vi "Taiko_TaggedValueListToStr.vi"(10 "TaggedValueList in":T1 {"Tag" format="%x" items=["NONE"=0, "Locked"=16, "SoftLock"=17, "KeyLock"=18, "Class_IV_Lock"=20, "Interlock"=24, "LaserMode"=32, "LDH_PulsePowerTable"=33, "TriggerMode"=48, "TriggerLevelRaw"=64, "TriggerLevelRawLoLimit"=65, "TriggerLevelRawHiLimit"=66, "TriggerLevel"=72, "TriggerLevelLoLimit"=73, "TriggerLevelHiLimit"=74, "FastGate"=80, "FastGateImp"=96, "SlowGate"=112, "TargetTempRaw"=144, "TargetTempRawLoLimit"=145, "TargetTempRawHiLimit"=146, "CurrentTempRaw"=148, "CaseTempRaw"=149, "TargetTemp"=152, "TargetTempLoLimit"=153, "TargetTempHiLimit"=154, "CurrentTemp"=156, "CaseTemp"=157, "TempScale"=159, "Frequency"=168, "FrequencyLoLimit"=169, "FrequencyHiLimit"=170, "PulsePowerRaw"=176, "PulsePowerRawLoLimit"=177, "PulsePowerRawHiLimit"=178, "PulsePowerPermille"=180, "PulseShape"=181, "PulsePower"=184, "PulsePowerLoLimit"=185, "PulsePowerHiLimit"=186, "PulsePowerNanowatt"=188, "PulsePowerVoltage"=190, "PulseEnergy"=191, "CwPowerRaw"=192, "CwPowerRawLoLimit"=193, "CwPowerRawHiLimit"=194, "CwPowerPermille"=196, "CwPower"=200, "CwPowerLoLimit"=201, "CwPowerHiLimit"=202, "CwPowerMicroWatt"=204, "BurstLen"=208, "BurstPeriod"=224, "LDH_Fan"=240, "UI_Exclusive"=256]}, 11 "String in":string) -> (3 "String out":string)   [LabVIEW 2019]
uses:
  <userlib>/TaikoLaser/PDLM_TaggedValueList.ctl
  <userlib>/TaikoLaser/PDLM_TaggedValue.ctl
  <userlib>/TaikoLaser/PDLM_Tag.ctl
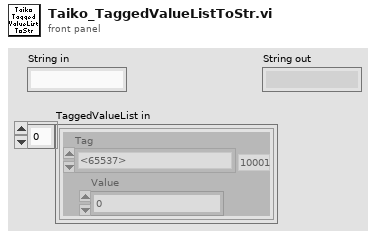
[diagram p1: front panel]
types:
  T1 = typedef "PDLM_TaggedValueList.ctl" = T2[]
  T2 = typedef "PDLM_TaggedValue.ctl" = cluster{"Tag":T3, "Value":u32}
  T3 = typedef "PDLM_Tag.ctl" = u32
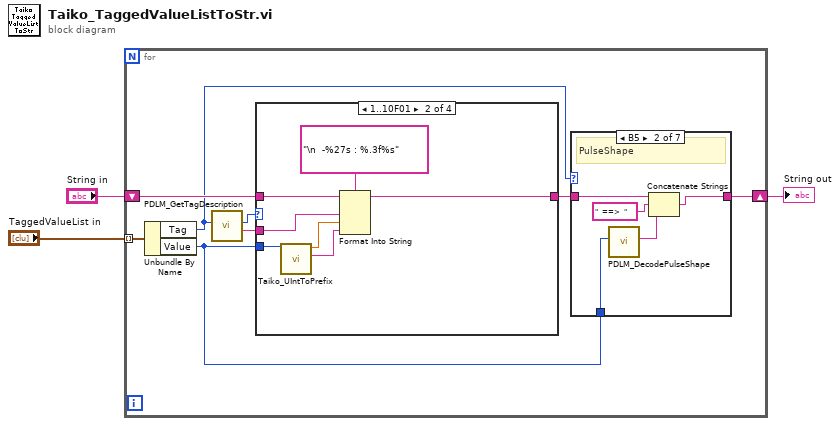
[diagram p0: block diagram]
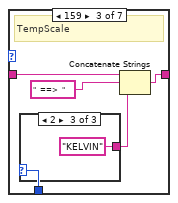
[diagram p3: hidden frame]
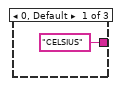
[diagram p4: hidden frame]
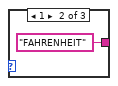
[diagram p5: hidden frame]
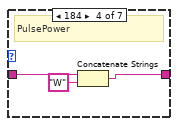
[diagram p6: hidden frame]
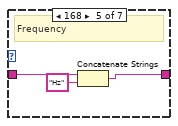
[diagram p7: hidden frame]
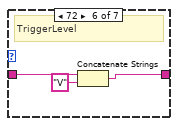
[diagram p8: hidden frame]
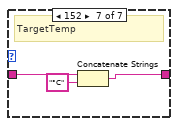
[diagram p9: hidden frame]
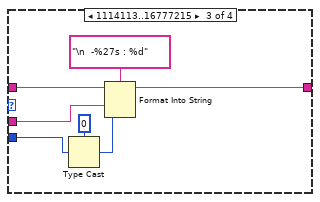
[diagram p11: hidden frame]
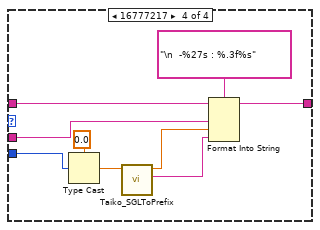
[diagram p12: hidden frame]
diagram:
  n1 = for {
    tunnel: "TaggedValueList in" -> [w11] mode=indexing
    shift-right: [w6] -> w2
    shift-left: "String in" -> [w9]
    n2 = Unbundle By Name(w11) -> ("Tag"=w4:T3, "Value"=w5:u32)
    n3 = call <userlib>:"PDLM_GetTagDescription.vi"("Tag"=w4) -> ("Name"=w10:string, "TypeCode"=w8:u32)  [unwired: 7 in, 2 out]
    n4 = case shown="1..10F01" w8 {
      tunnel: w10 -> [_ w45 w52 w61]
      tunnel: w5 -> [_ w41 w47 w56]
      tunnel: [w38 w39 w50 w59] -> w7
      tunnel: w9 -> [w38 w43 w49 w58]
      frame Default {
      }
      frame 1..69377 {
        n5 = call <userlib>:"Taiko_UIntToPrefix.vi"("UINT"=w41) -> ("PREFIX"=w40:string, "MANT"=w42:sgl)  [unwired: 9 in]
        n6 = Format Into String(format string="\n  -%27s : %.3f%s", initial string=w43, w45, w42, w40) -> (resulting string=w39:string)  [unwired: 1 in, 1 out]
      }
      frame 1114113..16777215 {
        n7 = Type Cast(type=0, x=w47) -> (*(type *) &x=w46:i32)
        n8 = Format Into String(format string="\n  -%27s : %d", initial string=w49, w52, w46) -> (resulting string=w50:string)  [unwired: 1 in, 1 out]
      }
      frame 16777217 {
        n9 = Type Cast(type=sgl 0.0, x=w56) -> (*(type *) &x=w55:sgl)
        n10 = call <userlib>:"Taiko_SGLToPrefix.vi"("SGL"=w55) -> ("PREFIX"=w53:string, "MANT"=w54:sgl)  [unwired: 9 in]
        n11 = Format Into String(format string="\n  -%27s : %.3f%s", initial string=w58, w61, w54, w53) -> (resulting string=w59:string)  [unwired: 1 in, 1 out]
      }
    }
    n12 = case shown="B5" w4 {
      tunnel: [w12 w16 w21 w27 w30 w33 w36] -> w6
      tunnel: w7 -> [w12 w17 w22 w28 w31 w34 w37]
      tunnel: w5 -> [_ w13 w19 _ _ _ _]
      frame Default {
      }
      frame 181 {
        # "PulseShape"
        n13 = call <userlib>:"PDLM_DecodePulseShape.vi"("shape"=w13) -> ("Buffer"=w15:string)  [unwired: 8 in, 2 out]
        n14 = Concatenate Strings(w17, "  ==>  " ("string"), w15) -> (w16:string)
      }
      frame 159 {
        # "TempScale"
        n15 = case shown="2" w19 {
          tunnel: ["CELSIUS" ("string") "FAHRENHEIT" ("string") "KELVIN" ("string")] -> w18
          frame 0, Default {
          }
          frame 1 {
          }
          frame 2 {
          }
        }
        n16 = Concatenate Strings(w22, "  ==>  " ("string"), w18) -> (w21:string)
      }
      frame 184 {
        # "PulsePower"
        n17 = Concatenate Strings(w28, "W" ("string")) -> (w27:string)
      }
      frame 168 {
        # "Frequency"
        n18 = Concatenate Strings(w31, "Hz" ("string")) -> (w30:string)
      }
      frame 72 {
        # "TriggerLevel"
        n19 = Concatenate Strings(w34, "V" ("string")) -> (w33:string)
      }
      frame 152 {
        # "TargetTemp"
        n20 = Concatenate Strings(w37, "°C" ("string")) -> (w36:string)
      }
    }
  }
  "String out" <- w2
